vi "ClearAll.vi"(8 "error in":errorcluster) -> (0 "error out":errorcluster)   [LabVIEW 2016]
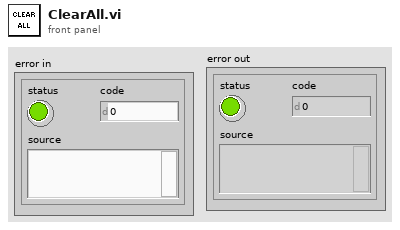
[diagram p1: front panel]
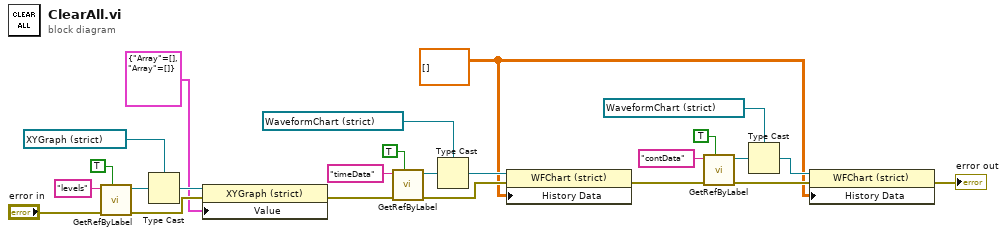
[diagram p0: block diagram]
diagram:
  w2 = dbl[][] [] ("History Data")
  n1 = call "GetRefByLabel.vi"("InsideTab"=TRUE, "error in"="error in", "Label"="levels") -> ("error out"=w20:errorcluster, "Ctl Refnum"=w22:refnum<vi>)  [unwired: 6 in, 1 out]
  n2 = Type Cast(type=refnum<vi> refnum ("levels"), x=w22) -> (*(type *) &x=w21:refnum<vi>)
  n3 = property class="XYGraph (strict)"(reference=w21, error in=w20, "Value"=cluster{"Array":i32[], "Array":dbl[]} {"Array"=[], "Array"=[]}) -> (error out=w17:errorcluster)  [unwired: 1 out]
  n4 = call "GetRefByLabel.vi"("InsideTab"=TRUE, "error in"=w17, "Label"="timeData") -> ("error out"=w15:errorcluster, "Ctl Refnum"=w14:refnum<vi>)  [unwired: 6 in, 1 out]
  n5 = Type Cast(type=refnum<vi> refnum ("timeData"), x=w14) -> (*(type *) &x=w13:refnum<vi>)
  n6 = property class="WFChart (strict)"(reference=w13, error in=w15, "History Data"=w2) -> (error out=w5:errorcluster)  [unwired: 1 out]
  n7 = call "GetRefByLabel.vi"("InsideTab"=TRUE, "error in"=w5, "Label"="contData") -> ("error out"=w4:errorcluster, "Ctl Refnum"=w8:refnum<vi>)  [unwired: 6 in, 1 out]
  n8 = Type Cast(type=refnum<vi> refnum ("timeData"), x=w8) -> (*(type *) &x=w3:refnum<vi>)
  n9 = property class="WFChart (strict)"(reference=w3, error in=w4, "History Data"=w2) -> (error out=→"error out":errorcluster)  [unwired: 1 out]
